vi "Configure.vi"(8 "error in":errorcluster, 10 "name":string, 11 "PAS in":refnum<class "PAS.lvclass">) -> (0 "error out":errorcluster, 3 "PAS out":refnum<class "PAS.lvclass">)   [LabVIEW 2014, in "PAS Library.lvlib" / "PAS.lvclass"]
doc: "Configure the instrument class. If there is no config file specified, an error"
uses:
  PAS.lvclass
  <vilib>/Utility/config.llb/NI_LVConfig.lvlib
  Session APIs/File Access/Config Data/Config Data.lvclass
  <vilib>/Utility/config.llb/Read Key (I32).vi
  Instrument/Instrument.lvclass
  <vilib>/Utility/config.llb/Read Key (Double).vi
  Data/Main/PAS Data.lvclass
  PAS/Commands/Load New Speaker Chirp/Load New Speaker Chirp.lvclass
  PAS/Commands/Change Speaker State/Change Speaker State.lvclass
  Data/Data.lvclass
  Cell/PAS Cell.lvclass
  Data/Cell/PAS Cell Data.lvclass
  <vilib>/Utility/config.llb/Read Key (Boolean).vi
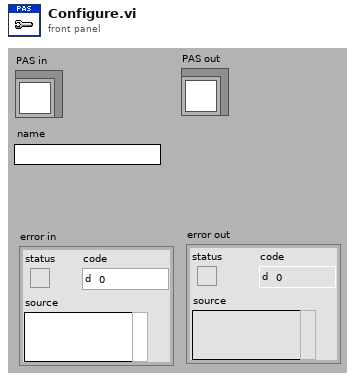
[diagram p1: front panel]
types:
  T1 = typedef "Config Data.lvclass/Config Session.ctl" = refnum<data-value>
  T2 = typedef "NI_LVConfig.lvlib/Config Data RefNum.ctl" = refnum<k1>
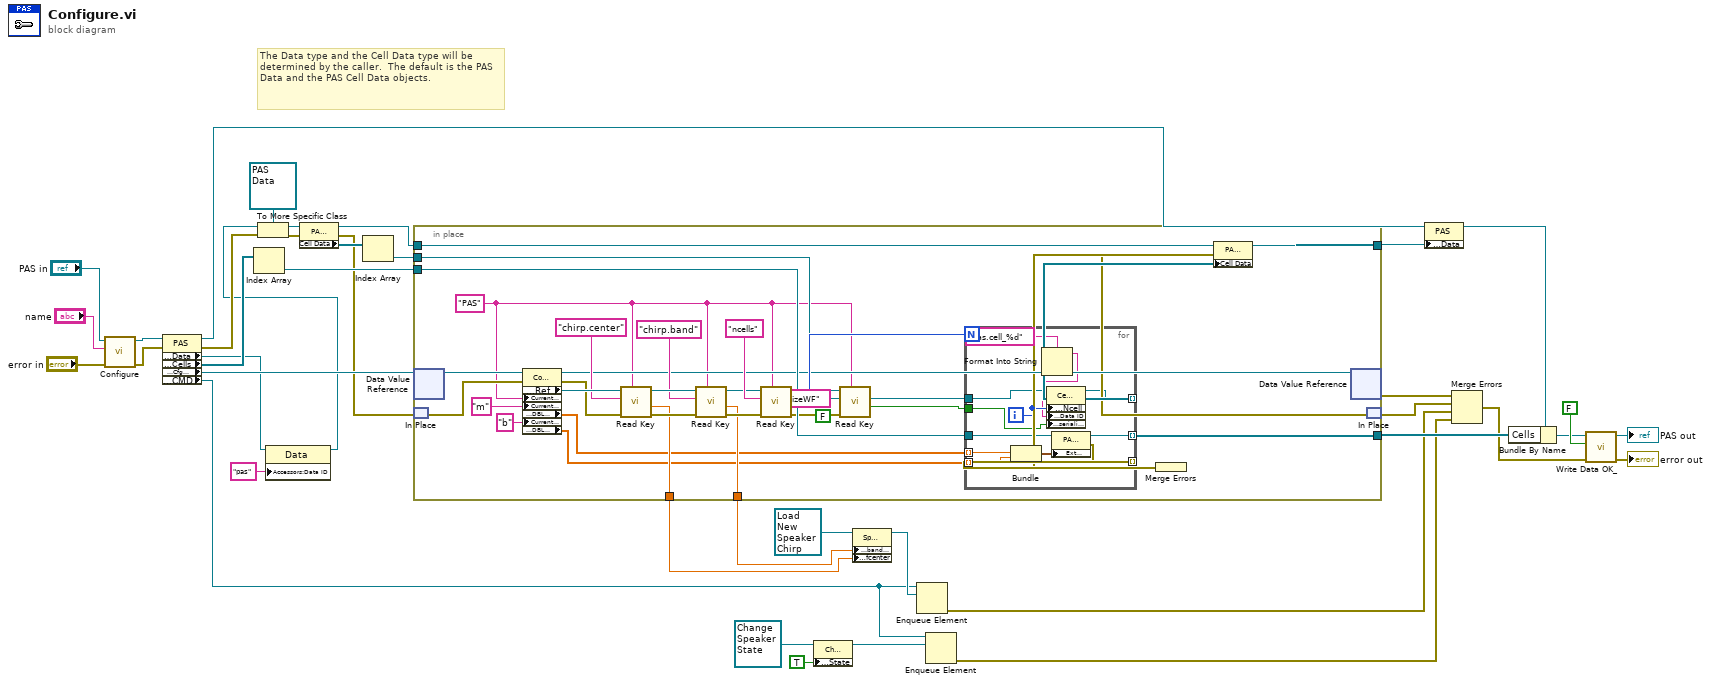
[diagram p0: block diagram]
diagram:
  # "The Data type and the Cell Data type will be determined by the caller.  The default is the PAS Data and the PAS Cell Data objects."
  n1 = call-parent "Configure.vi"("error in"="error in", "name"="name", "Instrument in"="PAS in") -> ("error out"=w36:errorcluster, "Instrument out"=w37:refnum<class "PAS.lvclass">)  [unwired: 7 in]
  n2 = property class="PAS"(reference=w37, error in=w36) -> (reference out=w26:refnum<class "PAS.lvclass">, error out=w14:errorcluster, "Accessors:Data"=w3:refnum<class "Data.lvclass">, "Data Access:Cells"=w15:refnum<class "PAS Cell.lvclass">[], "Accessors:Cfg Session"=w16:T1, "Accessors:CMD"=w7:refnum<queue>)
  n3 = Index Array(array=w15) -> (element=w35:refnum<class "PAS Cell.lvclass">)  [unwired: 1 in]
  n4 = property class="Data"(reference=w3, "Accessors:Data ID"="pas" ("Data ID")) -> (reference out=w2:refnum<class "Data.lvclass">)  [unwired: 1 in, 1 out]
  n5 = To More Specific Class(target class=refnum<class "PAS Data.lvclass"> refnum ("PAS Data"), reference=w2, error in=w14) -> (specific class reference=w24:refnum<class "PAS Data.lvclass">, error out=w13:errorcluster)
  n6 = property class="PAS Data"(reference=w24, error in=w13) -> (reference out=w21:refnum<class "PAS Data.lvclass">, error out=w12:errorcluster, "Cell Data"=w23:refnum<class "PAS Cell Data.lvclass">[])
  n7 = Index Array(array=w23) -> (element=w22:refnum<class "PAS Cell Data.lvclass">)  [unwired: 1 in]
  n8 = in-place {
    in-place-border: w35 -> [w71]
    in-place-border: [w70] -> w34
    in-place-border: [w66] -> w27
    in-place-border: w22 -> [w58]
    in-place-border: w21 -> [w57]
    in-place-border: [w56] -> w19
    in-place-border: [w55] -> w18
    w45 = "PAS" ("section")
    n9 = in-place-dvr #1(w16) -> (w74:refnum<class "Config Data.lvclass">)  [unwired: 1 out]
    n10 = in-place-match #2(w12) -> (w69:errorcluster)
    n11 = property class="Config Data"(reference=w74, error in=w69, "Current Section"=w45, "Current Key"="m", "Current Key"="b") -> (reference out=w49:refnum<class "Config Data.lvclass">, error out=w61:errorcluster, "Accessors:Ref"=w65:T2, "Read Array Data:DBL Data"=w51:dbl[], "Read Array Data:DBL Data"=w50:dbl[])
    n12 = call-poly <vilib>:"Read Key.vi"("section"=w45, "error in (no error)"=w61, "key"="chirp.center", "refnum"=w65) -> ("error out"=w60:errorcluster, "value"=w55:dbl, "refnum out"=w64:T2)  [unwired: 4 in, 1 out]
    n13 = call-poly <vilib>:"Read Key.vi"("section"=w45, "error in (no error)"=w60, "key"="chirp.band", "refnum"=w64) -> ("error out"=w59:errorcluster, "value"=w56:dbl, "refnum out"=w54:T2)  [unwired: 4 in, 1 out]
    n14 = call-poly <vilib>:"Read Key.vi"("section"=w45, "error in (no error)"=w59, "key"="ncells", "refnum"=w54) -> ("error out"=w43:errorcluster, "value"=w72:i32, "refnum out"=w46:T2)  [unwired: 4 in, 1 out]
    n15 = call-poly <vilib>:"Read Key.vi"("section"=w45, "error in (no error)"=w43, "default value"=FALSE, "key"="serializeWF", "refnum"=w46) -> ("value"=w42:bool)  [unwired: 3 in, 3 out]
    n16 = for {
      N: w72 -> [_]
      tunnel: w71 -> [w86]
      tunnel: [w85] -> w70 mode=indexing
      tunnel: [w84] -> w68 mode=indexing
      tunnel: [w79] -> w67 mode=indexing
      tunnel: w58 -> [w80]
      tunnel: w51 -> [w83] mode=indexing
      tunnel: w50 -> [w82] mode=indexing
      tunnel: w42 -> [w75]
      i -> [w78]
      n17 = Bundle(w83, w82) -> (w81:cluster{dbl, dbl})  [unwired: 1 in]
      n18 = Format Into String(format string="pas.cell_%d", w78) -> (resulting string=w76:string)  [unwired: 2 in, 1 out]
      n19 = property class="Cell Data"(reference=w80, "Accessors:Ncell"=w78, "Accessors:Data ID"=w76, "Accessors:serializeWF_"=w75) -> (reference out=w79:refnum<class "PAS Cell Data.lvclass">)  [unwired: 1 in, 1 out]
      n20 = property class="PAS Cell"(reference=w86, "Ext Params"=w81) -> (reference out=w85:refnum<class "PAS Cell.lvclass">, error out=w84:errorcluster)  [unwired: 1 in]
    }
    n21 = Merge Errors(w68) -> (w48:errorcluster)
    n22 = property class="PAS Data"(reference=w57, error in=w48, "Cell Data"=w67) -> (reference out=w66:refnum<class "PAS Data.lvclass">, error out=w47:errorcluster)
    n23 = in-place-dvr #1(w49) -> (w32:errorcluster)  [unwired: 1 out]
    n24 = in-place-match #2(w47) -> (w33:errorcluster)
  }
  n25 = property class="Change Speaker State"(reference=refnum<class "Change Speaker State.lvclass"> refnum ("Change Speaker State"), "Accessors:State"=TRUE ("State")) -> (reference out=w8:refnum<class "Change Speaker State.lvclass">)  [unwired: 1 in, 1 out]
  n26 = property class="Speaker Chirp"(reference=refnum<class "Load New Speaker Chirp.lvclass"> refnum ("Speaker Chirp"), "Accessors:bandwidth"=w19, "Accessors:fcenter"=w18) -> (reference out=w17:refnum<class "Load New Speaker Chirp.lvclass">)  [unwired: 1 in, 1 out]
  n27 = Enqueue Element(queue=w7, element=w17) -> (error out=w6:errorcluster)  [unwired: 2 in, 2 out]
  n28 = Enqueue Element(queue=w7, element=w8) -> (error out=w5:errorcluster)  [unwired: 2 in, 2 out]
  n29 = property class="PAS"(reference=w26, "Accessors:Data"=w27) -> (reference out=w28:refnum<class "PAS.lvclass">)  [unwired: 1 in, 1 out]
  n30 = Merge Errors(w32, w33, w6, w5) -> (w4:errorcluster)
  n31 = Bundle By Name(cluster=w28, "Cells"=w34) -> (w29:refnum<class "PAS.lvclass">)
  n32 = call "Write Data OK_.vi"("error in (no error)"=w4, "Data OK?"=FALSE ("goodData"), "Instrument in"=w29) -> ("error out"=→"error out":errorcluster, "Instrument out"=→"PAS out":refnum<class "PAS.lvclass">)  [unwired: 7 in]
